vi "Brk_Pt_Triggers.vi"(0 "Board ID":T3=1 min=1 max=32 step=1, 1 "Axis":T1=1 items=["Axis 1"=1, "Axis 2"=2, "Axis 3"=3, "Axis 4"=4, "Axis 5"=5, "Axis 6"=6, "Axis 7"=7, "Axis 8"=8], 2 "Reverse ?":bool, 5 "Number of steps":i32=10, 9 "Step interval":i32=1, 11 "error in (no error)":errorcluster, 12 "Total steps":i32) -> (4 "Start Position":i32, 6 "End Position":i32, 10 "Motion error":bool)   [LabVIEW 2022 SP3]
doc: "EXAMPLE: DO_WHILE Loop (Onboard Programming Template)\n\nSUMMARY:\nThis FlexMotion example demonstrates the implementation of a DO_WHILE loop data structure in an onboard program. The C equivalent of the data structure implemented here is:\n\ndo {\n// code to be repeated\nloopVar = loopVar - increment;\n} while (loopVar != 0);\n\nTHEORY OF OPERATION:\nThe flow of the DO_WHILE loop data structure goes as follows:\n(1) Program storage is begun.\n(2) The DO_WHILE loop is set up. (Loop Variable and Increment are each defined and initialized.)\n(3) A code delimiter is set using label #1.\n(4) Code to be executed each time through loop is run (in the template program, the loop variable is decremented).\n(5) The loop variable or other test condition is checked.\n(6) If the test condition is true, then we jump back to label #1. Otherwise, the condition is false so the loop terminates.\n(7) Program storage is ended.\n\nDEVELOPMENT DETAILS:\nApplication Software: LabVIEW 5.0.x\nHardware: FlexMotion controller\nDriver Software: FlexMotion Software 4.0\n\nREQUIRED HARDWARE:\n(controller only)\n\nINSTRUCTIONS:\n(0) Initialize the FlexMotion controller before running this VI. \n(1) Add the FlexMotion functions you want to execute into the block diagram where noted.\n(2) Run the VI to store the program. (The program will not be executed at this time.)\n(3) You can then run the program you have stored by calling the run_prog.flx function with the appropriate program number.\n\nADDITIONAL NOTES:\n(a) You should read the following items before writing FlexMotion onboard programs:\n(1) The Onboard Programs section of the FlexMotion Hardware User Manual (page 4-9 in the November 1998 edition).\n(2) The section about onboard variables in your FlexMotion Software Reference Manual (pages 4-11 and 4-12 in the November 1998 edition)\n(3) You will find the chapter of the FlexMotion Software Reference Manual concerning the Onboard Programming functions to be an invaluable reference resource (Chapter 12 of the November 1998 edition) along with the online help for the VI functions.\n(b) This template repeats the DO_WHILE loop as long as an expression with a variable evaluates to be true. However, you may evaluate other conditions such as move complete status instead.\n\n*NOTE: This example is not supported on the 7334 controller."
uses:
  <vilib>/Motion/FlexMotion/FunctionsVIs/AnalogDigitalIO.llb/Set I/O Port MOMO.flx
  -MotionRoutines/MotionGlobals.vi
  <vilib>/Motion/FlexMotion/FunctionsVIs/StartStopMotion.llb/Start Motion (8 axes).flx
  <vilib>/Motion/FlexMotion/FunctionsVIs/MotionIO.llb/Set Breakpoint Output MOMO (6 axes).flx
  <vilib>/Motion/FlexMotion/FunctionsVIs/Trajectory.llb/Load Acceleration/Deceleration.flx
  <vilib>/Motion/FlexMotion/CustomControls/CustomControls.llb/Buffer.flx
  <vilib>/Motion/FlexMotion/CustomControls/CustomControls.llb/Program.flx
  <vilib>/Motion/FlexMotion/CustomControls/CustomControls.llb/Axis To Read.flx
panel:
  in  "Case Constant\n(See Context Help)":bool
  out "Done loop":i32
  out "Motion stop loop":i32
  in  "Program (1)":T2=1 format="%.0x"
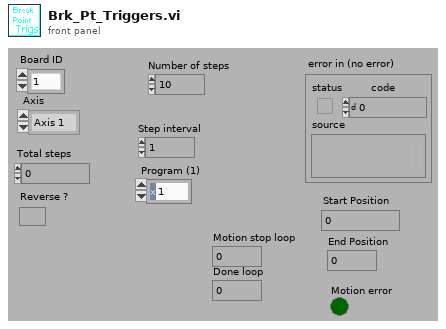
[diagram p1: front panel]
types:
  T1 = typedef "Axis To Read.flx" = u16
  T2 = typedef "Program.flx" = u8
  T3 = typedef "Board Id" = u8
  T4 = enum16{"General-Purpose Input", "General-Purpose Output", "Position", "Breakpoint Data", "High-Speed Capture Readback"}
  T5 = typedef "Buffer.flx" = u8
  T6 = enum16{"No Change", "Reset on Breakpoint", "Set on Breakpoint", "Toggle on Breakpoint", "Create Pulse on Breakpoint"}
  T7 = enum16{"Absolute Breakpoint", "Relative Breakpoint", "Modulo Breakpoint", "Periodic Breakpoint"}
  T8 = enum16{"Single Breakpoint", "Buffered Breakpoint"}
  T9 = typedef "Bd Id Out" = u8
  T10 = cluster{"1":bool, "2":bool, "3":bool, "4":bool, "5":bool, "6":bool}
  T11 = typedef "MustOn" = cluster{"0":bool, "1":bool, "2":bool, "3":bool, "4":bool, "5":bool, "6":bool, "7":bool}
  T12 = typedef "Resource Out (Enum).flx" = u16
  T13 = enum16{"Less Than", "Equal", "Less Than Or Equal", "Greater Than", "Not Equal", "Greater Than Or Equal", "True", "Home Found", "Index Found", "High Speed Capture", "Position Breakpoint", "Reserved", "Velocity Threshold", "Move Complete", "Profile Complete", "Blend Complete", "Motor Off", "Home Input Active", "Limit Input Active", "Software Limit Active", "Program Complete", "IO Port Match"}
  T14 = typedef "Buffer Out.flx" = u8
  T15 = enum16{"Buffer Not Exist", "Ready", "Active", "Done", "Old Data Stop"}
  T16 = cluster{"Reserved":bool, "Axis #1 Move Complete":bool, "Axis #2 Move Complete":bool, "Axis #3 Move Complete":bool, "Axis #4 Move Complete":bool, "Axis #5 Move Complete":bool, "Axis #6 Move Complete":bool, "Axis #7 Move Complete":bool, "Axis #8 Move Complete":bool, "Axis #9 MoveComplete":bool, "Axis #10 Move Complete":bool, "Axis #11 Move Complete":bool, "Axis #12 Move Complete":bool, "Status #13":bool, "Status #14":bool, "Status #15":bool}
  T17 = cluster{"Run/Stop":bool, "Profile Complete":bool, "Motor Off ":bool, "Following Error":bool, "Limit Switch":bool, "Home Switch":bool, "SW Limit Switch":bool, "Watchdog":bool, "Velocity Threshold":bool, "Position Brkpt":bool, "Home Found":bool, "Index Found":bool, "High Speed Capture":bool, "Reverse Direction":bool, "Blend Complete":bool, "Move Complete":bool}
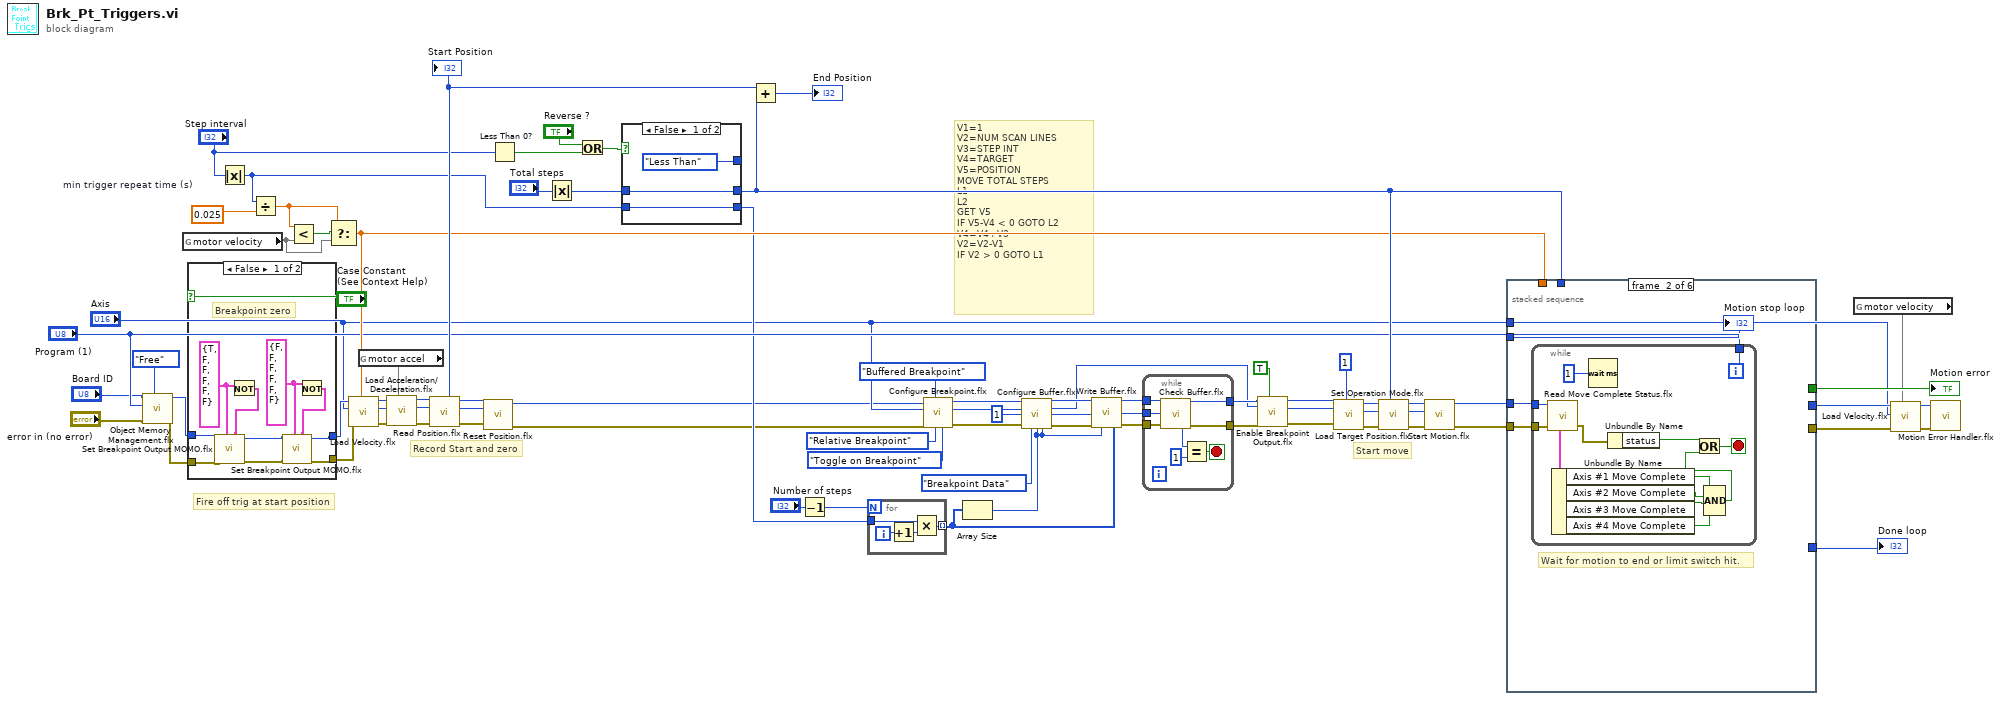
[diagram p0: block diagram]
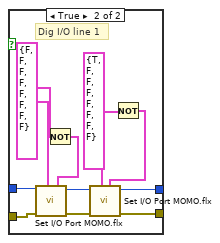
[diagram p2: hidden frame]
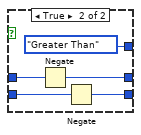
[diagram p3: hidden frame]
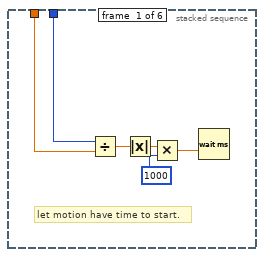
[diagram p4: hidden frame]
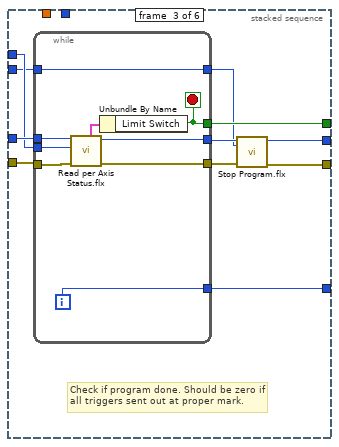
[diagram p5: hidden frame]
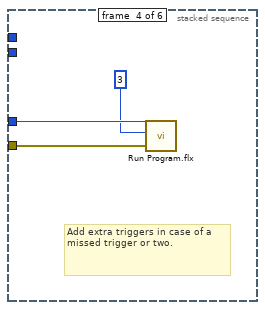
[diagram p6: hidden frame]
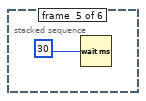
[diagram p7: hidden frame]
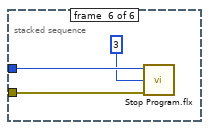
[diagram p8: hidden frame]
diagram:
  w61 = 0.025  # min trigger repeat time (s)
  # "Fire off trig at start position"
  # "V1=1\nV2=NUM SCAN LINES\nV3=STEP INT\nV4=TARGET\nV5=POSITION\nMOVE TOTAL STEPS\nL1\nL2\nGET V5\nIF V5-V4 < 0 GOTO L2\nV4=V4+V3\nV2=V2-V1\nIF V2 > 0 GOTO L1"
  # "Record Start and zero"
  # "Start move"
  n1 = call <vilib>:"Object Memory Management.flx"("Operation"=enum16{"Save", "Delete", "Free"}."Free" ("Operation (Free)"), "error in (no error)"="error in (no error)", "Object (1)"="Program (1)", "Board ID"="Board ID") -> ("error out"=w35:errorcluster, "Bd ID Out"=w32:T9)  [unwired: 4 out]
  n2 = global read "MotionGlobals.vi" "motor velocity"() -> (w46)
  n3 = case shown="False" "Case Constant\n(See Context Help)" {
    tunnel: [w81 w97] -> w33
    tunnel: [w80 w96] -> w34
    tunnel: w32 -> [w85 w92]
    tunnel: w35 -> [w84 w94]
    frame False {
      w86 = T10 {"1"=TRUE, "2"=FALSE, "3"=FALSE, "4"=FALSE, "5"=FALSE, "6"=FALSE} ("Must On")
      w88 = T10 {"1"=FALSE, "2"=FALSE, "3"=FALSE, "4"=FALSE, "5"=FALSE, "6"=FALSE} ("Must On")
      # "Breakpoint zero"
      n4 = Not(x=w86) -> (.not. x?=w87:T10)
      n5 = call-poly <vilib>:"Set Breakpoint Output MOMO.flx"("Must Off"=w87, "Must On"=w86, "error in (no error)"=w84, "Board ID"=w85) -> ("error out"=w82:errorcluster, "Bd ID Out"=w83:T9)  [unwired: 2 in, 2 out]
      n6 = Not(x=w88) -> (.not. x?=w89:T10)
      n7 = call-poly <vilib>:"Set Breakpoint Output MOMO.flx"("Must Off"=w89, "Must On"=w88, "error in (no error)"=w82, "Board ID"=w83) -> ("error out"=w80:errorcluster, "Bd ID Out"=w81:T9)  [unwired: 2 in, 2 out]
    }
    frame True {
      w98 = T11 {"0"=TRUE, "1"=FALSE, "2"=FALSE, "3"=FALSE, "4"=FALSE, "5"=FALSE, "6"=FALSE, "7"=FALSE} ("Must On")
      w99 = T11 {"0"=FALSE, "1"=FALSE, "2"=FALSE, "3"=FALSE, "4"=FALSE, "5"=FALSE, "6"=FALSE, "7"=FALSE} ("Must On")
      # "Dig I/O line 1"
      n8 = Not(x=w99) -> (.not. x?=w91:T11)
      n9 = call "Set I/O Port MOMO.flx"("Must Off"=w91, "Must On"=w99, "error in (no error)"=w94, "Board ID"=w92) -> ("error out"=w95:errorcluster, "Bd ID Out"=w93:T9)  [unwired: 2 in, 2 out]
      n10 = Not(x=w98) -> (.not. x?=w90:T11)
      n11 = call "Set I/O Port MOMO.flx"("Must Off"=w90, "Must On"=w98, "error in (no error)"=w95, "Board ID"=w93) -> ("error out"=w96:errorcluster, "Bd ID Out"=w97:T9)  [unwired: 2 in, 2 out]
    }
  }
  n12 = Absolute Value(x="Step interval") -> (abs(x)=w49:i32)
  n13 = Divide(x=w49, y=w61) -> (x/y=w59:dbl)
  n14 = Less?(x=w59, y=w46) -> (x < y?=w60:bool)
  n15 = Select(t=w59, s=w60, f=w46) -> (s? t:f=w56:dbl)
  n16 = call <vilib>:"Load Velocity.flx"("Velocity (10000)"=w56, "error in (no error)"=w34, "Axis or Vector Space"="Axis", "Board ID"=w33) -> ("error out"=w42:errorcluster, "Resource Output"=w39:T12, "Bd ID Out"=w41:T9)  [unwired: 3 out]
  n17 = global read "MotionGlobals.vi" "motor accel"() -> (w40)
  n18 = call "Load Acceleration/Deceleration.flx"("Acceleration (100000)"=w40, "error in (no error)"=w42, "Axis or Vector Space"=w39, "Board ID"=w41) -> ("error out"=w43:errorcluster, "Resource Output"=w36:T12, "Bd ID Out"=w44:T9)  [unwired: 1 in, 2 out]
  n19 = call <vilib>:"Read Position.flx"("error in (no error)"=w43, "Axis"=w36, "Board ID"=w44) -> ("error out"=w72:errorcluster, "Resource Output"=w71:T12, "Bd ID Out"=w73:T9, "Position"=w67:i32)  [unwired: 3 out]
  "Start Position" <- w67
  n20 = call <vilib>:"Reset Position.flx"("error in (no error)"=w72, "Axis"=w71, "Board ID"=w73) -> ("error out"=w3:errorcluster, "Bd ID Out"=w4:T9)  [unwired: 2 in, 3 out]
  n21 = Less Than 0?(x="Step interval") -> (x < 0?=w53:bool)
  n22 = Absolute Value(x="Total steps") -> (abs(x)=w51:i32)
  n23 = Or(x="Reverse ?", y=w53) -> (x .or. y?=w50:bool)
  n24 = case shown="False" w50 {
    tunnel: w51 -> [w102 w107]
    tunnel: [w102 w106] -> w66
    tunnel: [w101 w104] -> w24
    tunnel: w49 -> [w101 w105]
    tunnel: [T13."Less Than" ("Condition Code (True)") T13."Greater Than" ("Condition Code (True)")] -> _
    frame False {
    }
    frame True {
      n25 = Negate(x=w107) -> (-x=w106:i32)
      n26 = Negate(x=w105) -> (-x=w104:i32)
    }
  }
  n27 = Add(x=w67, y=w66) -> (x+y=→"End Position":i32)
  n28 = Decrement(x="Number of steps") -> (x-1=w25:i32)
  n29 = for {
    N: w25 -> [_]
    tunnel: w24 -> [w110]
    tunnel: [w109] -> w22 mode=indexing
    i -> [w111]
    n30 = Increment(x=w111) -> (x+1=w108:i32)
    n31 = Multiply(x=w110, y=w108) -> (x*y=w109:i32)
  }
  n32 = call <vilib>:"Configure Breakpoint.flx"("Action (No Change)"=T6."Toggle on Breakpoint", "Mode (Absolute)"=T7."Relative Breakpoint", "Operation (Single)"=T8."Buffered Breakpoint", "error in (no error)"=w3, "Axis or Encoder"="Axis", "Board ID"=w4) -> ("error out"=w19:errorcluster, "Resource Output"=w10:T12, "Bd ID Out"=w20:T9)  [unwired: 3 out]
  n33 = Array Size(array=w22) -> (size(s)=w7:i32)
  n34 = call <vilib>:"Configure Buffer.flx"("Board ID"=w20, "Resource"=w10, "Buffer"=T5 1, "error in (no error)"=w19, "Buffer Type (Position)"=T4."Breakpoint Data", "Buffer Size"=w7, "Total Points"=w7) -> ("Bd ID Out"=w27:T9, "Resource Output"=w5:T12, "Buffer Out"=w13:T14, "error out"=w26:errorcluster)  [unwired: 2 in, 3 out]
  n35 = call <vilib>:"Write Buffer.flx"("Board ID"=w27, "Buffer"=w13, "error in (no error)"=w26, "Number of Points (0)"=w7, "Data"=w22) -> ("Bd ID Out"=w15:T9, "Buffer Out"=w16:T14, "error out"=w14:errorcluster)  [unwired: 1 in, 7 out]
  n36 = while {
    tunnel: w16 -> [w119]
    tunnel: w15 -> [w118]
    tunnel: w14 -> [w117]
    tunnel: [w116] -> w12
    tunnel: [w115] -> w11
    stop <- w112 stop-if-true
    n37 = call <vilib>:"Check Buffer.flx"("Board ID"=w118, "Buffer"=w119, "error in (no error)"=w117) -> ("Bd ID Out"=w115:T9, "Buffer  State"=w114:T15, "error out"=w116:errorcluster)  [unwired: 10 out]
    n38 = Equal?(x=w114, y=1) -> (x = y?=w112:bool)
  }
  n39 = call <vilib>:"Enable Breakpoint Output.flx"("Enable Breakpoint"=TRUE, "error in (no error)"=w12, "Axis or Encoder"=w5, "Board ID"=w11) -> ("error out"=w9:errorcluster, "Resource Output"=w6:T12, "Bd ID Out"=w8:T9)  [unwired: 3 out]
  n40 = call <vilib>:"Set Operation Mode.flx"("Position Mode (Absolute)"=1, "error in (no error)"=w9, "Axis or Vector Space"=w6, "Board ID"=w8) -> ("error out"=w76:errorcluster, "Resource Output"=w70:T12, "Bd ID Out"=w77:T9)  [unwired: 2 out]
  n41 = call <vilib>:"Load Target Position.flx"("Target Position (0)"=w66, "error in (no error)"=w76, "Axis"=w70, "Board ID"=w77) -> ("error out"=w78:errorcluster, "Resource Output"=w79:T12, "Bd ID Out"=w74:T9)  [unwired: 3 out]
  n42 = call-poly <vilib>:"Start Motion.flx"("error in (no error)"=w78, "Axis or Vector Space"=w79, "Board ID"=w74) -> ("error out"=w1:errorcluster, "Bd ID Out"=w2:T9)  [unwired: 1 in, 3 out]
  n43 = stacked-sequence {
    tunnel: w2 -> [_ w128 w152 w164 _ w168]
    tunnel: w1 -> [_ w126 w151 w163 _ w167]
    tunnel: w66 -> [w122 _ _ _ _ _]
    tunnel: [_ _ w150 _ _ _] -> w64
    tunnel: [_ _ w149 _ _ _] -> w63
    tunnel: w56 -> [w120 _ _ _ _ _]
    tunnel: "Axis" -> [_ _ w148 _ _ _]
    tunnel: "Program (1)" -> [_ _ w147 _ _ _]
    tunnel: [_ _ w146 _ _ _] -> w48
    tunnel: [_ _ w145 _ _ _] -> w47
    frame #0 {
      # "let motion have time to start."
      n44 = Divide(x=w122, y=w120) -> (x/y=w123:dbl)
      n45 = Absolute Value(x=w123) -> (abs(x)=w124:dbl)
      n46 = Multiply(x=w124, y=1000) -> (x*y=w121:dbl)
      n47 = Wait (ms)(milliseconds to wait=w121) -> ()  [unwired: 1 out]
    }
    frame #1 {
      # "Wait for motion to end or limit switch hit."
      n48 = while {
        tunnel: w128 -> [w141]
        tunnel: [w130] -> w127
        tunnel: w126 -> [w129]
        i -> [w130]
        stop <- w132 stop-if-true
        n49 = call <vilib>:"Read Move Complete Status.flx"("error in (no error)"=w129, "Board ID"=w141) -> ("error out"=w140:errorcluster, "Move Complete Status"=w139:T16)  [unwired: 1 in, 4 out]
        n50 = Unbundle By Name(w139) -> ("Axis #1 Move Complete"=w135:bool, "Axis #2 Move Complete"=w138:bool, "Axis #3 Move Complete"=w137:bool, "Axis #4 Move Complete"=w136:bool)
        n51 = Wait (ms)(milliseconds to wait=1) -> ()  [unwired: 1 out]
        n52 = Unbundle By Name(w140) -> ("status"=w134:bool)
        n53 = Compound Arithmetic op=AND(w135, w138, w137, w136) -> (w133:bool)
        n54 = Or(x=w134, y=w133) -> (x .or. y?=w132:bool)
      }
      "Motion stop loop" <- w127
    }
    frame #2 {
      # "Check if program done. Should be zero if all triggers sent out at proper mark."
      n55 = while {
        tunnel: w151 -> [w158]
        tunnel: [w161] -> w143
        tunnel: [w160] -> w144
        tunnel: w152 -> [w159]
        tunnel: [w153] -> w150
        tunnel: [w157] -> w149
        tunnel: w148 -> [w156]
        tunnel: w147 -> [w155]
        tunnel: [w155] -> w142
        i -> [w157]
        stop <- w153 stop-if-true
        n56 = call <vilib>:"Read per Axis Status.flx"("error in (no error)"=w158, "Axis"=w156, "Board ID"=w159) -> ("error out"=w160:errorcluster, "Bd ID Out"=w161:T9, "Per Axis H/W Status"=w154:T17)  [unwired: 4 out]
        n57 = Unbundle By Name(w154) -> ("Limit Switch"=w153:bool)
      }
      n58 = call <vilib>:"Stop Program.flx"("error in (no error)"=w144, "Program (1)"=w142, "Board ID"=w143) -> ("error out"=w145:errorcluster, "Bd ID Out"=w146:T9)  [unwired: 4 out]
    }
    frame #3 {
      # "Add extra triggers in case of a missed trigger or two."
      n59 = call <vilib>:"Run Program.flx"("error in (no error)"=w163, "Program (1)"=3, "Board ID"=w164) -> ()  [unwired: 6 out]
    }
    frame #4 {
      n60 = Wait (ms)(milliseconds to wait=30) -> ()  [unwired: 1 out]
    }
    frame #5 {
      n61 = call <vilib>:"Stop Program.flx"("error in (no error)"=w167, "Program (1)"=3, "Board ID"=w168) -> ()  [unwired: 6 out]
    }
  }
  "Motion error" <- w64
  "Done loop" <- w63
  n62 = global read "MotionGlobals.vi" "motor velocity"() -> (w57)
  n63 = call <vilib>:"Load Velocity.flx"("Velocity (10000)"=w57, "error in (no error)"=w47, "Axis or Vector Space"="Axis", "Board ID"=w48) -> ("error out"=w45:errorcluster, "Bd ID Out"=w58:T9)  [unwired: 4 out]
  n64 = call <vilib>:"Motion Error Handler.flx"("Board ID"=w58, "error in (no error)"=w45) -> ()  [unwired: 3 in, 11 out]
